vi "VerticalSettings.vi"(5 "Channel B":T1={"Enable"=FALSE, "Vertical coupling"=0, "Vertical range"=0.0, "Vertical offset"=0.0, "Probe attenuation"=1.0}, 7 "Channel A":T1={"Enable"=FALSE, "Vertical coupling"=0, "Vertical range"=0.0, "Vertical offset"=0.0, "Probe attenuation"=1.0}, 8 "error in":errorcluster {"code" format="%.0x"}, 11 "instrument handle":refnum<k15>) -> (0 "error out":errorcluster {"code" format="%.0x"}, 1 "Vertical range Channel B":dbl, 2 "Vertical range Channel A":dbl, 3 "instrument handle out":refnum<k15>)   [LabVIEW 2011]
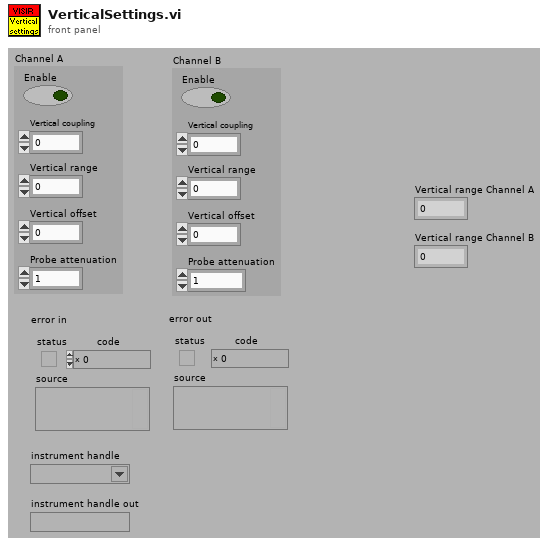
[diagram p1: front panel]
types:
  T1 = cluster{"Enable":bool, "Vertical coupling":i32, "Vertical range":dbl, "Vertical offset":dbl, "Probe attenuation":dbl}
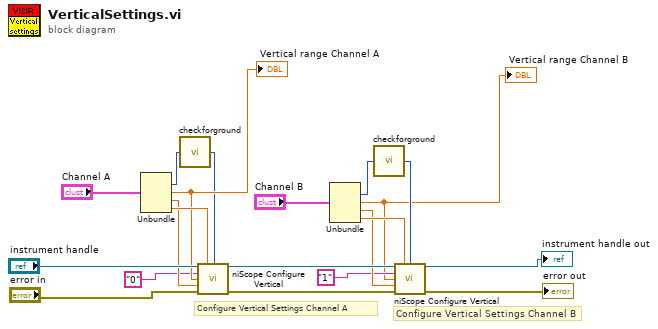
[diagram p0: block diagram]
diagram:
  # "Configure Vertical Settings Channel B"
  # "Configure Vertical Settings Channel A"
  n1 = Unbundle("Channel A") -> ("Vertical coupling"=w5:i32, "Vertical range"=w11:dbl, "Vertical offset"=w12:dbl, "Probe attenuation"=w13:dbl)  [unwired: 1 out]
  "Vertical range Channel A" <- w11
  n2 = call "checkforground.vi"("Vertical coupling"=w5) -> ("If GND; set in AC mode (GND mode will be fixed later)"=w4:i32)
  n3 = call <instrlib>:"niScope Configure Vertical.vi"("instrument handle"="instrument handle", "probe attenuation"=w13, "vertical coupling"=w4, "channels"="0" ("channel name"), "vertical range"=w11, "vertical offset"=w12, "error in"="error in") -> ("instrument handle out"=w14:refnum<k15>, "error out"=w17:errorcluster)  [unwired: 7 in]
  n4 = Unbundle("Channel B") -> ("Vertical coupling"=w3:i32, "Vertical range"=w1:dbl, "Vertical offset"=w8:dbl, "Probe attenuation"=w9:dbl)  [unwired: 1 out]
  "Vertical range Channel B" <- w1
  n5 = call "checkforground.vi"("Vertical coupling"=w3) -> ("If GND; set in AC mode (GND mode will be fixed later)"=w2:i32)
  n6 = call <instrlib>:"niScope Configure Vertical.vi"("instrument handle"=w14, "probe attenuation"=w9, "vertical coupling"=w2, "channels"="1" ("channel name"), "vertical range"=w1, "vertical offset"=w8, "error in"=w17) -> ("instrument handle out"=→"instrument handle out":refnum<k15>, "error out"=→"error out":errorcluster)  [unwired: 7 in]
